vi "get_error_text.vi"(11 "Код ошибки":i16) -> (0 "Событие":string, 3 "Механизм":string)   [LabVIEW 2011]
panel:
  out "Array 2":string[](array[string])
  out "Array":string[](array[string])
  out "floor(x/y)":i16 format="%x"
  out "x-y*floor(x/y)":i16 format="%x"
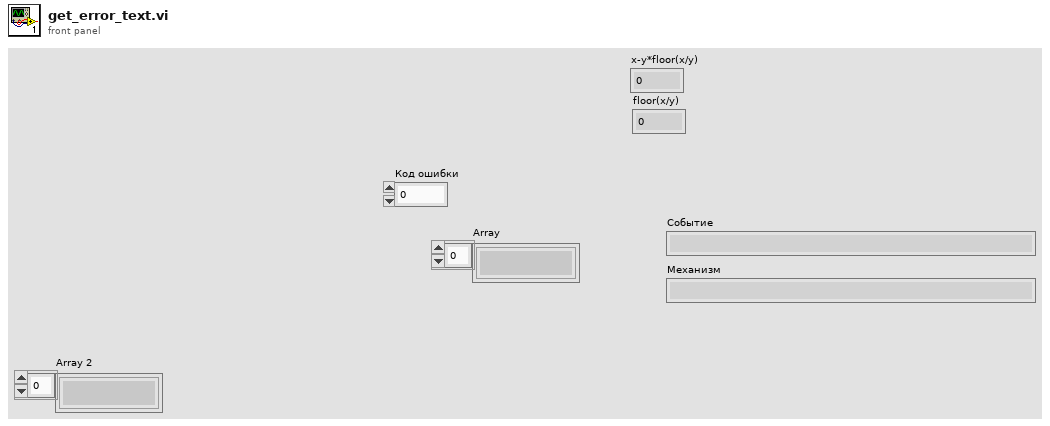
[diagram p1: front panel]
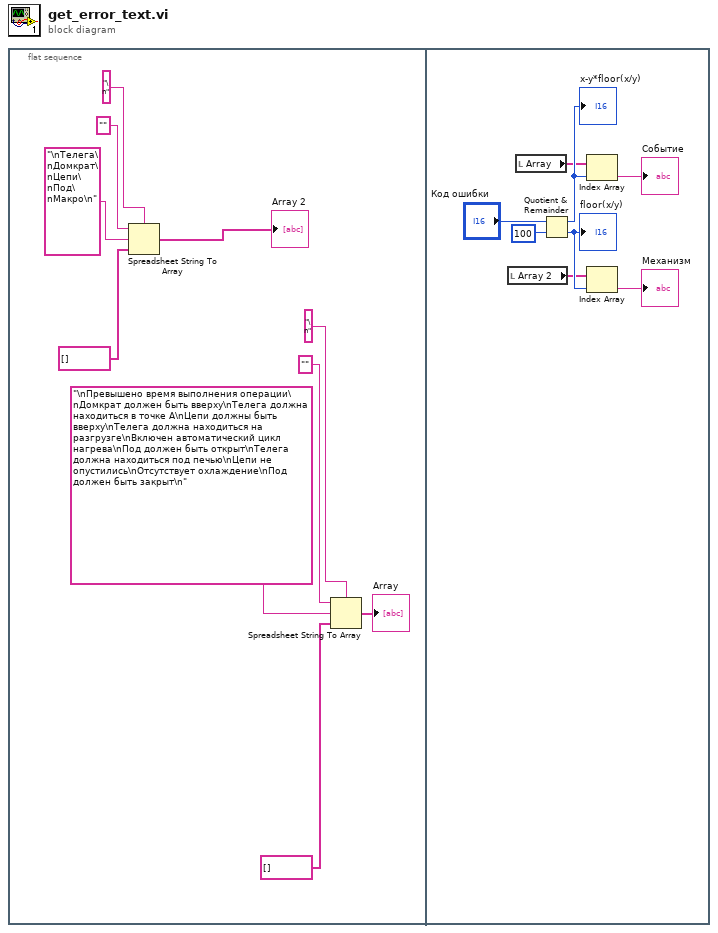
[diagram p0: block diagram]
diagram:
  n1 = flat-sequence {
    frame #0 {
      n2 = Spreadsheet String To Array(delimiter (Tab)="\n", format string="", spreadsheet string="\nТелега\nДомкрат\nЦепи\nПод\nМакро\n", array type (2D Dbl)=string[] [] ("ОП1 Х1")) -> (array=→"Array 2":string[])
      n3 = Spreadsheet String To Array(delimiter (Tab)="\n", format string="", spreadsheet string="\nПревышено время выполнения операции\nДомкрат должен быть вверху\nТелега должна находиться в точке А\nЦепи должны быть вверху\nТелега должна находиться на разгрузге\nВключен автоматический цикл нагрева\nПод должен быть открыт\nТелега должна находиться под печью\nЦепи не опустились\nОтсутствует охлаждение\nПод должен быть закрыт\n", array type (2D Dbl)=string[] [] ("ОП1 Х1")) -> (array=→"Array":string[])
    }
    frame #1 {
      n4 = local read "Array 2"() -> (w12:string[])
      n5 = local read "Array"() -> (w11:string[])
      n6 = Quotient & Remainder(x="Код ошибки", y=i16 100) -> (x-y*floor(x/y)=w13:i16, floor(x/y)=w16:i16)
      "x-y*floor(x/y)" <- w13
      "floor(x/y)" <- w16
      n7 = Index Array(array=w11, index=w13) -> (element=→"Событие":string)
      n8 = Index Array(array=w12, index=w16) -> (element=→"Механизм":string)
    }
  }
